vi "Data cluster.vi"() -> ()   [LabVIEW 2010, in "SQL project lib.lvlib"]
uses:
  SQL project lib.lvlib
panel:
  out "output cluster":T1
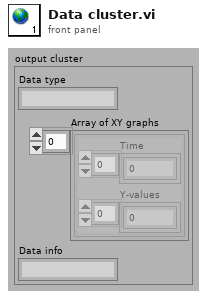
[diagram p1: front panel]
types:
  T1 = cluster{"Data type":string, "Array of XY graphs":cluster{"Time":dbl[], "Y-values":dbl[]}[], "Data info":string}
diagram:
